vi "update_dust_event_small.vi"(8 "error in (no error)":errorcluster, 11 "Cluster":T1 {"File Location" items=["Unknown"=-1, "Storage"=0, "Processing"=1]}) -> (0 "error out":errorcluster)   [LabVIEW 2015]
uses:
  User Interface/Controls/Post_Dust_Event_small.ctl
  User Interface/Controls/File_location.ctl
panel:
  # "Dust Event Small"
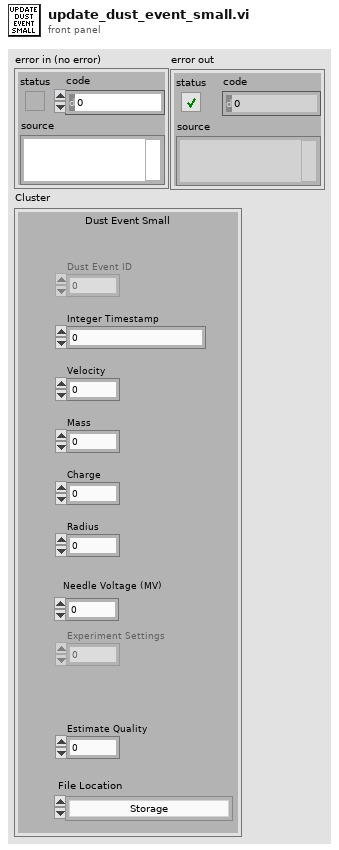
[diagram p1: front panel]
types:
  T1 = typedef "Post_Dust_Event_small.ctl" = cluster{"Dust Event ID":i64, "Integer Timestamp":i64, "Velocity":sgl, "Mass":sgl, "Charge":sgl, "Radius":sgl, "Needle Voltage (MV)":dbl, "Experiment Settings":dbl, "Estimate Quality":sgl, "File Location":T2, "id_dust_info":dbl}
  T2 = typedef "File_location.ctl" = i8
  T3 = cluster{"Velocity":sgl, "Mass":sgl, "Charge":sgl, "Radius":sgl, "Estimate Quality":sgl, "File Location":T2}
  T4 = cluster{"Velocity":string, "Mass":string, "Charge":string, "Radius":string, "Estimate Quality":string, string}
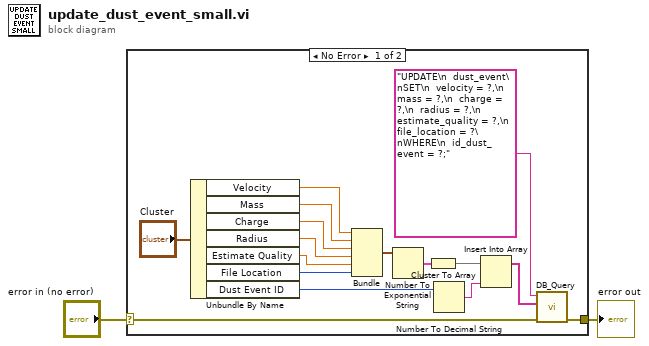
[diagram p0: block diagram]
diagram:
  n1 = case shown="No Error" "error in (no error)" {
    selector: "error in (no error)" -> [w6 w19]
    tunnel: [w5 w19] -> w1
    frame No Error {
      n2 = Unbundle By Name("Cluster") -> ("Velocity"=w14:sgl, "Mass"=w18:sgl, "Charge"=w17:sgl, "Radius"=w16:sgl, "Estimate Quality"=w15:sgl, "File Location"=w13:T2, "Dust Event ID"=w3:i64)
      n3 = Bundle("Velocity"=w14, "Mass"=w18, "Charge"=w17, "Radius"=w16, "Estimate Quality"=w15, "File Location"=w13) -> (w4:T3)  [unwired: 1 in]
      n4 = Number To Exponential String(number=w4) -> (E-format string=w7:T4)  [unwired: 3 in]
      n5 = Cluster To Array(cluster=w7) -> (array=w10:string[])
      n6 = Number To Decimal String(number=w3) -> (decimal integer string=w11:string)  [unwired: 1 in]
      n7 = Insert Into Array(array=w10, new element=w11) -> (w9:string[])  [unwired: 1 in]
      n8 = call "DB_Query.vi"("error in (no error)"=w6, "Parameters"=w9, "Parameterized Query"="UPDATE\n  dust_event\nSET\n  velocity = ?,\n  mass = ?,\n  charge = ?,\n  radius = ?,\n  estimate_quality = ?,\n  file_location = ?\nWHERE\n  id_dust_event = ?;") -> ("error out"=w5:errorcluster)  [unwired: 6 in, 2 out]
    }
    frame Error {
    }
  }
  "error out" <- w1
